vi "dfd_Maxflat Find Polynomial.vi"(4 "H0":dbl, 6 "x0":dbl=0.49999999999999994, 8 "error in (no error)":errorcluster, 9 "N":i32=2, 10 "M":i32=1, 11 "L":i32=3) -> (0 "error out":errorcluster, 1 "c":dbl, 2 "denominator":dbl[](array[numeric]), 3 "numerator":dbl[](array[numeric]) format="%_10g")   [LabVIEW 2017, in "NI_DigFilter_Design.lvlib"]
doc: "Founds the polynomial for calculating the coefficients of the filter."
uses:
  <vilib>/addons/Digital Filter Design/NI_DigFilter_Design.lvlib
  <vilib>/addons/Digital Filter Design/_Misc.llb/dfd_Error Cluster From Error Code (Scalar).vi
  <vilib>/addons/Digital Filter Design/NI_DigFilter_Process.lvlib
  <vilib>/addons/Digital Filter Design/NI_DigFilterLicensed.lvlib
  <vilib>/Analysis/NI_AALBase.lvlib
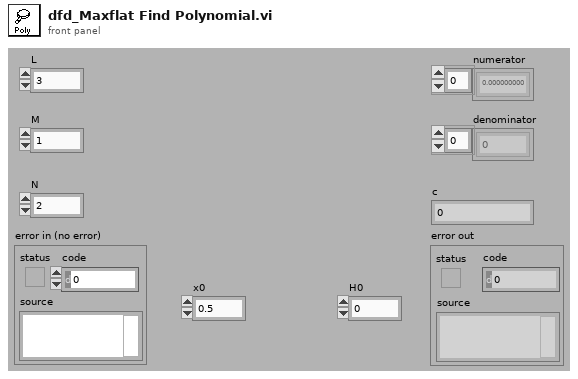
[diagram p1: front panel]
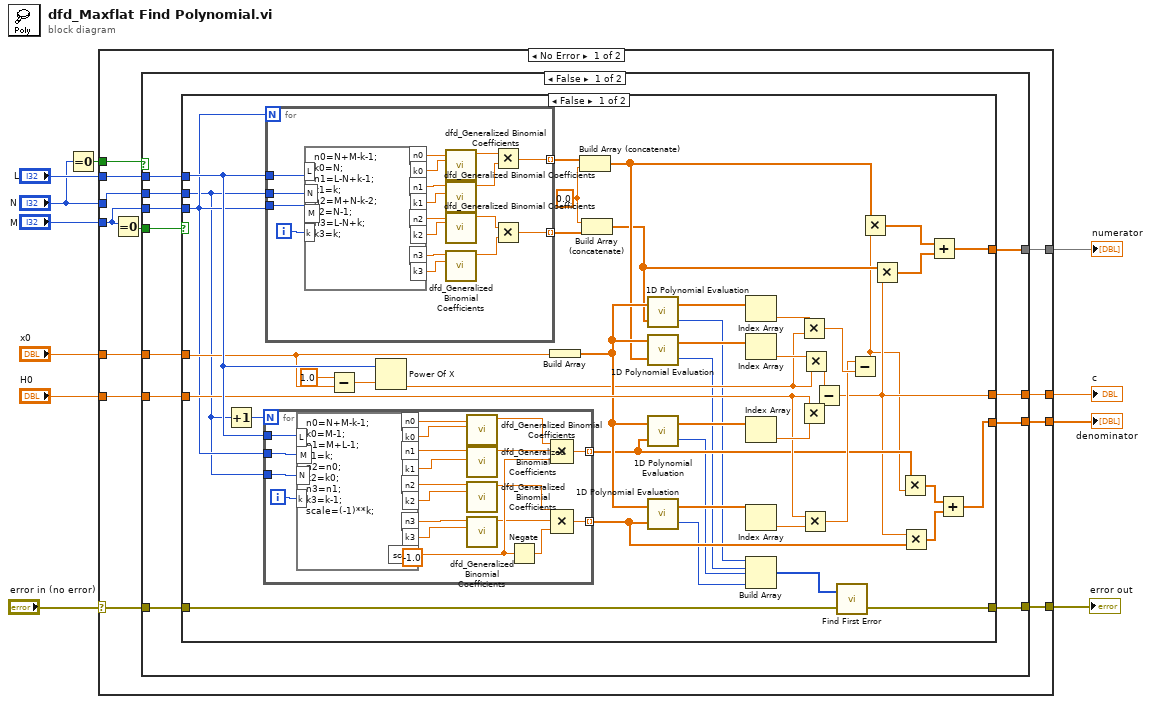
[diagram p0: block diagram]
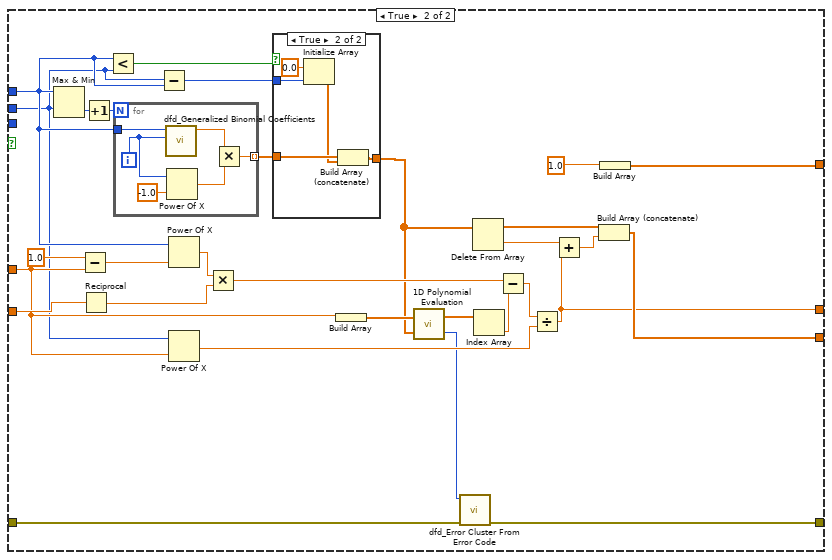
[diagram p2: hidden frame]
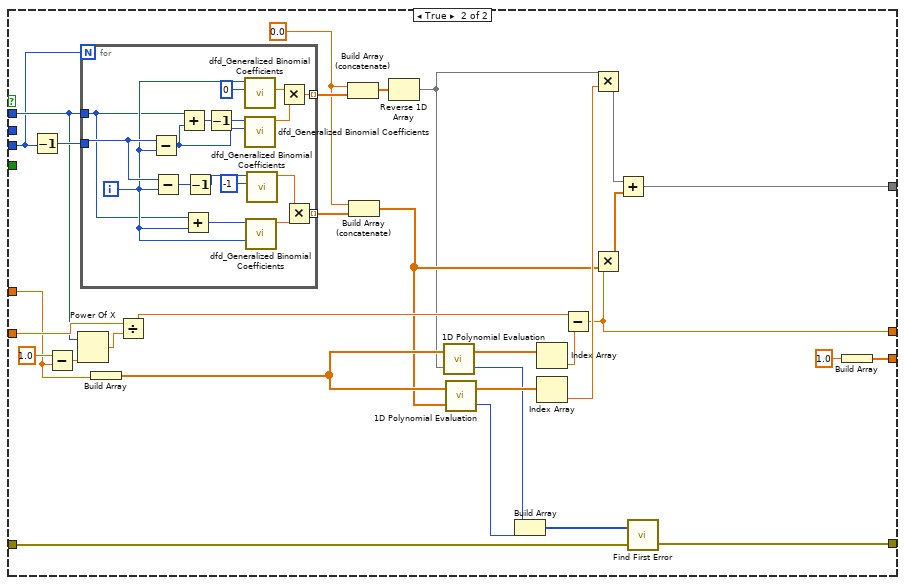
[diagram p4: hidden frame]
diagram:
  n1 = Equal To 0?(x="N") -> (x = 0?=w1:bool)
  n2 = case shown="No Error" "error in (no error)" {
    selector: "error in (no error)" -> [w13 w207]
    tunnel: "M" -> [w22 _]
    tunnel: "H0" -> [w21 _]
    tunnel: "x0" -> [w20 _]
    tunnel: "N" -> [w19 _]
    tunnel: "L" -> [w18 _]
    tunnel: [w17 _] -> w7
    tunnel: [w16 _] -> w6
    tunnel: [w15 w207] -> w4
    tunnel: [w14 _] -> w3
    tunnel: w1 -> [w12 _]
    frame No Error {
      n3 = Equal To 0?(x=w22) -> (x = 0?=w23:bool)
      n4 = case shown="False" w12 {
        tunnel: w23 -> [w34 _]
        tunnel: w18 -> [w32 w185]
        tunnel: w19 -> [w31 _]
        tunnel: w22 -> [w27 w170]
        tunnel: w20 -> [w30 w168]
        tunnel: w21 -> [w29 w188]
        tunnel: [w33 w175] -> w17
        tunnel: [w28 w174] -> w16
        tunnel: [w26 w172] -> w15
        tunnel: w13 -> [w25 w169]
        tunnel: [w24 w171] -> w14
        frame False {
          n5 = case shown="False" w34 {
            tunnel: [w45 w145] -> w33
            tunnel: w32 -> [w76 w138]
            tunnel: w31 -> [w49 w129]
            tunnel: w30 -> [w75 w130]
            tunnel: w29 -> [w66 w137]
            tunnel: [w53 w122] -> w28
            tunnel: w27 -> [w50 _]
            tunnel: w25 -> [w36 w118]
            tunnel: [w37 w117] -> w26
            tunnel: [w52 w120] -> w24
            frame False {
              w46 = 0.0
              n6 = Increment(x=w49) -> (x+1=w51:i32)
              n7 = for {
                N: w51 -> [_]
                tunnel: w76 -> [w82]
                tunnel: [w97] -> w55 mode=indexing
                tunnel: [w94] -> w54 mode=indexing
                tunnel: w50 -> [w81]
                tunnel: w49 -> [w80]
                i -> [w79]
                (unwired) -1.0 ("x")
                n8 = formula code="n0=N+M-k-1;\nk0=M-1;\nn1=M+L-1;\nk1=k;\nn2=n0;\nk2=k0;\nn3=n1;\nk3=k-1;\nscale=(-1)**k;"("N"=w80, "M"=w81, "k"=w79, "L"=w82) -> ("n0"=w92:dbl, "k0"=w91:dbl, "n1"=w90:dbl, "k1"=w89:dbl, "n2"=w88:dbl, "k2"=w87:dbl, "n3"=w86:dbl, "k3"=w85:dbl, "scale"=w93:dbl)
                n9 = call <vilib>:"dfd_Generalized Binomial Coefficients.vi"("k"=w91, "n"=w92) -> ("binomial coefficient (n,k)"=w95:dbl)  [unwired: 1 in, 8 out]
                n10 = call <vilib>:"dfd_Generalized Binomial Coefficients.vi"("k"=w89, "n"=w90) -> ("binomial coefficient (n,k)"=w98:dbl)  [unwired: 1 in, 8 out]
                n11 = call <vilib>:"dfd_Generalized Binomial Coefficients.vi"("k"=w87, "n"=w88) -> ("binomial coefficient (n,k)"=w83:dbl)  [unwired: 1 in, 8 out]
                n12 = call <vilib>:"dfd_Generalized Binomial Coefficients.vi"("k"=w85, "n"=w86) -> ("binomial coefficient (n,k)"=w84:dbl)  [unwired: 1 in, 8 out]
                n13 = Negate(x=w93) -> (-x=w96:dbl)
                n14 = Compound Arithmetic op=MULTIPLY(w95, w98, w93) -> (w97:dbl)
                n15 = Compound Arithmetic op=MULTIPLY(w83, w84, w96) -> (w94:dbl)
              }
              n16 = for {
                N: w50 -> [_]
                tunnel: w50 -> [w111]
                tunnel: w76 -> [w110]
                tunnel: w49 -> [w109]
                tunnel: [w100] -> w47 mode=indexing
                tunnel: [w99] -> w48 mode=indexing
                i -> [w112]
                n17 = formula code="n0=N+M-k-1;\nk0=N;\nn1=L-N+k-1;\nk1=k;\nn2=M+N-k-2;\nk2=N-1;\nn3=L-N+k;\nk3=k;"("N"=w109, "M"=w111, "k"=w112, "L"=w110) -> ("n0"=w108:dbl, "k0"=w107:dbl, "n1"=w106:dbl, "k1"=w105:dbl, "n2"=w104:dbl, "k2"=w103:dbl, "n3"=w102:dbl, "k3"=w101:dbl)
                n18 = call <vilib>:"dfd_Generalized Binomial Coefficients.vi"("k"=w107, "n"=w108) -> ("binomial coefficient (n,k)"=w116:dbl)  [unwired: 1 in, 8 out]
                n19 = call <vilib>:"dfd_Generalized Binomial Coefficients.vi"("k"=w105, "n"=w106) -> ("binomial coefficient (n,k)"=w115:dbl)  [unwired: 1 in, 8 out]
                n20 = call <vilib>:"dfd_Generalized Binomial Coefficients.vi"("k"=w103, "n"=w104) -> ("binomial coefficient (n,k)"=w114:dbl)  [unwired: 1 in, 8 out]
                n21 = call <vilib>:"dfd_Generalized Binomial Coefficients.vi"("k"=w101, "n"=w102) -> ("binomial coefficient (n,k)"=w113:dbl)  [unwired: 1 in, 8 out]
                n22 = Multiply(x=w116, y=w115) -> (x*y=w100:dbl)
                n23 = Multiply(x=w114, y=w113) -> (x*y=w99:dbl)
              }
              n24 = Subtract(x=1.0, y=w75) -> (x-y=w77:dbl)
              n25 = Power Of X(1:w77, 2:w76) -> (0:w62:dbl)
              n26 = Build Array(w75) -> (w64:dbl[])
              n27 = Build Array (concatenate)(w47, w46) -> (w44:dbl[])
              n28 = Build Array (concatenate)(w46, w48) -> (w43:dbl[])
              n29 = call <vilib>:"1D Polynomial Evaluation.vi"("Coefficients: a"=w43, "X"=w64) -> ("error"=w41:i32, "Y"=w65:dbl[])
              n30 = call <vilib>:"1D Polynomial Evaluation.vi"("Coefficients: a"=w44, "X"=w64) -> ("error"=w40:i32, "Y"=w74:dbl[])
              n31 = call <vilib>:"1D Polynomial Evaluation.vi"("Coefficients: a"=w55, "X"=w64) -> ("error"=w39:i32, "Y"=w72:dbl[])
              n32 = call <vilib>:"1D Polynomial Evaluation.vi"("Coefficients: a"=w54, "X"=w64) -> ("error"=w38:i32, "Y"=w67:dbl[])
              n33 = Index Array(array=w65) -> (element=w63:dbl)  [unwired: 1 in]
              n34 = Index Array(array=w74) -> (element=w73:dbl)  [unwired: 1 in]
              n35 = Index Array(array=w72) -> (element=w71:dbl)  [unwired: 1 in]
              n36 = Index Array(array=w67) -> (element=w68:dbl)  [unwired: 1 in]
              n37 = Build Array(w41, w40, w39, w38) -> (w35:i32[])
              n38 = Multiply(x=w63, y=w62) -> (x*y=w61:dbl)
              n39 = Multiply(x=w66, y=w71) -> (x*y=w69:dbl)
              n40 = Multiply(x=w66, y=w68) -> (x*y=w56:dbl)
              n41 = Multiply(x=w73, y=w62) -> (x*y=w70:dbl)
              n42 = Subtract(x=w70, y=w69) -> (x-y=w52:dbl)
              n43 = call <vilib>:"Find First Error.vi"("error in (no error)"=w36, "error codes"=w35) -> ("error out"=w37:errorcluster)  [unwired: 1 in, 2 out]
              n44 = Subtract(x=w56, y=w61) -> (x-y=w42:dbl)
              n45 = Multiply(x=w44, y=w42) -> (x*y=w60:dbl[])
              n46 = Multiply(x=w43, y=w52) -> (x*y=w59:dbl[])
              n47 = Multiply(x=w55, y=w42) -> (x*y=w57:dbl[])
              n48 = Multiply(x=w52, y=w54) -> (x*y=w58:dbl[])
              n49 = Add(x=w60, y=w59) -> (x+y=w45:dbl[])
              n50 = Add(x=w57, y=w58) -> (x+y=w53:dbl[])
            }
            frame True {
              n51 = Max & Min(x=w138, y=w129) -> (min(x,y)=w144:i32)  [unwired: 1 out]
              n52 = Subtract(x=1.0, y=w130) -> (x-y=w139:dbl)
              n53 = Reciprocal(x=w137) -> (1/x=w135:dbl)
              n54 = Increment(x=w144) -> (x+1=w119:i32)
              n55 = Less?(x=w138, y=w129) -> (x < y?=w143:bool)
              n56 = for {
                N: w119 -> [_]
                tunnel: w138 -> [w158]
                tunnel: [w153] -> w141 mode=indexing
                i -> [w156]
                n57 = call <vilib>:"dfd_Generalized Binomial Coefficients.vi"("k"=w156, "n"=w158) -> ("binomial coefficient (n,k)"=w155:dbl)  [unwired: 1 in, 8 out]
                n58 = Power Of X(1:-1.0 ("x"), 2:w156) -> (0:w154:dbl)
                n59 = Multiply(x=w155, y=w154) -> (x*y=w153:dbl)
              }
              n60 = Subtract(x=w129, y=w138) -> (x-y=w142:i32)
              n61 = Power Of X(1:w139, 2:w138) -> (0:w136:dbl)
              n62 = Power Of X(1:w130, 2:w129) -> (0:w127:dbl)
              n63 = Multiply(x=w136, y=w135) -> (x*y=w133:dbl)
              n64 = case shown="True" w143 {
                tunnel: w142 -> [_ w152]
                tunnel: w141 -> [w147 w150]
                tunnel: [w147 w148] -> w126
                frame False {
                }
                frame True {
                  n65 = Initialize Array(0.0 ("element"), w152) -> (w149:dbl[])
                  n66 = Build Array (concatenate)(w150, w149) -> (w148:dbl[])
                }
              }
              n67 = Build Array(w130) -> (w134:dbl[])
              n68 = call <vilib>:"1D Polynomial Evaluation.vi"("Coefficients: a"=w126, "X"=w134) -> ("error"=w121:i32, "Y"=w132:dbl[])
              n69 = call-poly <vilib>:"dfd_Error Cluster From Error Code.vi"("error in (no error)"=w118, "error code (0)"=w121) -> ("error out"=w117:errorcluster)  [unwired: 9 out]
              n70 = Delete From Array(array=w126) -> (deleted portion=w125:dbl, array with subset deleted=w124:dbl[])  [unwired: 2 in]
              n71 = Index Array(array=w132) -> (element=w131:dbl)  [unwired: 1 in]
              n72 = Subtract(x=w133, y=w131) -> (x-y=w128:dbl)
              n73 = Divide(x=w128, y=w127) -> (x/y=w120:dbl)
              n74 = Add(x=w125, y=w120) -> (x+y=w123:dbl)
              n75 = Build Array (concatenate)(w124, w123) -> (w122:dbl[])
              n76 = Build Array(1.0) -> (w145:dbl[])
            }
          }
        }
        frame True {
          w161 = 0.0 ("element")
          n77 = Decrement(x=w170) -> (x-1=w189:i32)
          n78 = Subtract(x=1.0, y=w168) -> (x-y=w184:dbl)
          n79 = Power Of X(1:w184, 2:w185) -> (0:w186:dbl)
          n80 = for {
            N: w170 -> [_]
            tunnel: w189 -> [w199]
            tunnel: w185 -> [w195]
            tunnel: [w191] -> w164 mode=indexing
            tunnel: [w190] -> w162 mode=indexing
            i -> [w196]
            n81 = Subtract(x=w199, y=w196) -> (x-y=w203:i32)
            n82 = Subtract(x=w199, y=w196) -> (x-y=w198:i32)
            n83 = Add(x=w195, y=w203) -> (x+y=w205:i32)
            n84 = Add(x=w195, y=w196) -> (x+y=w194:i32)
            n85 = Decrement(x=w198) -> (x-1=w197:i32)
            n86 = Decrement(x=w205) -> (x-1=w204:i32)
            n87 = call <vilib>:"dfd_Generalized Binomial Coefficients.vi"("k"=0, "n"=w196) -> ("binomial coefficient (n,k)"=w202:dbl)  [unwired: 1 in, 8 out]
            n88 = call <vilib>:"dfd_Generalized Binomial Coefficients.vi"("k"=w203, "n"=w204) -> ("binomial coefficient (n,k)"=w201:dbl)  [unwired: 1 in, 8 out]
            n89 = call <vilib>:"dfd_Generalized Binomial Coefficients.vi"("k"=w196, "n"=w194) -> ("binomial coefficient (n,k)"=w192:dbl)  [unwired: 1 in, 8 out]
            n90 = call <vilib>:"dfd_Generalized Binomial Coefficients.vi"("k"=-1, "n"=w197) -> ("binomial coefficient (n,k)"=w193:dbl)  [unwired: 1 in, 8 out]
            n91 = Multiply(x=w202, y=w201) -> (x*y=w190:dbl)
            n92 = Multiply(x=w193, y=w192) -> (x*y=w191:dbl)
          }
          n93 = Build Array(w168) -> (w180:dbl[])
          n94 = Divide(x=w188, y=w186) -> (x/y=w183:dbl)
          n95 = Build Array (concatenate)(w161, w162) -> (w160:dbl[])
          n96 = Build Array (concatenate)(w161, w164) -> (w163:dbl[])
          n97 = Reverse 1D Array(array=w160) -> (reversed array=w159:dbl[])
          n98 = call <vilib>:"1D Polynomial Evaluation.vi"("Coefficients: a"=w159, "X"=w180) -> ("error"=w167:i32, "Y"=w182:dbl[])
          n99 = call <vilib>:"1D Polynomial Evaluation.vi"("Coefficients: a"=w163, "X"=w180) -> ("error"=w166:i32, "Y"=w179:dbl[])
          n100 = Build Array(w167, w166) -> (w165:i32[])
          n101 = Index Array(array=w182) -> (element=w181:dbl)  [unwired: 1 in]
          n102 = Index Array(array=w179) -> (element=w178:dbl)  [unwired: 1 in]
          n103 = Subtract(x=w183, y=w181) -> (x-y=w171:dbl)
          n104 = Multiply(x=w159, y=w178) -> (x*y=w177:dbl[])
          n105 = Multiply(x=w163, y=w171) -> (x*y=w176:dbl[])
          n106 = Add(x=w177, y=w176) -> (x+y=w175:dbl[])
          n107 = call <vilib>:"Find First Error.vi"("error in (no error)"=w169, "error codes"=w165) -> ("error out"=w172:errorcluster)  [unwired: 1 in, 2 out]
          n108 = Build Array(1.0 ("element")) -> (w174:dbl[])
        }
      }
    }
    frame Error {
    }
  }
  "numerator" <- w7
  "denominator" <- w6
  "error out" <- w4
  "c" <- w3
